vi "List Path Configurations.vi"(8 "error in (no error)":errorcluster, 11 "VISA resource name":refnum<visa-resource-name>) -> (0 "error out":errorcluster, 2 "Path Configuration Array":string[](array[string]), 3 "VISA resource name out":refnum<visa-resource-name>)   [LabVIEW 2018, in "Keysight PNA Series.lvlib"]
doc: "Returns a list of configuration names stored in the PNA."
uses:
  Keysight PNA Series.lvlib
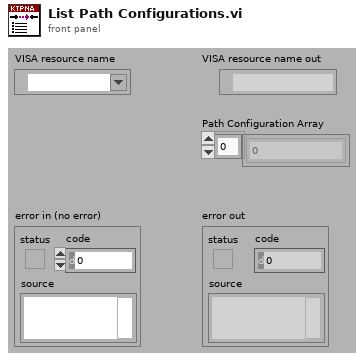
[diagram p1: front panel]
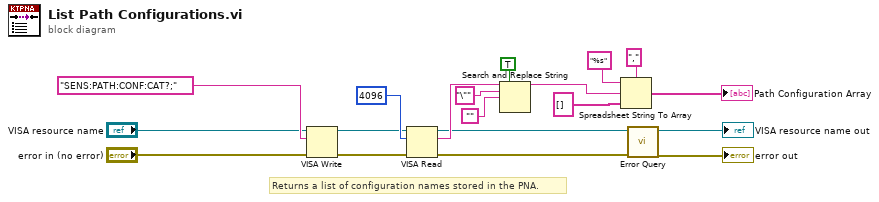
[diagram p0: block diagram]
diagram:
  # "Returns a list of configuration names stored in the PNA."
  n1 = VISA Write(VISA resource name="VISA resource name", write buffer="SENS:PATH:CONF:CAT?;", error in (no error)="error in (no error)") -> (VISA resource name out=w15:refnum<visa-resource-name>, error out=w14:errorcluster)  [unwired: 1 out]
  n2 = VISA Read(VISA resource name=w15, byte count=u32 4096, error in (no error)=w14) -> (VISA resource name out=w2:refnum<visa-resource-name>, read buffer=w3:string, error out=w4:errorcluster)  [unwired: 1 out]
  n3 = Search and Replace String(replace all?=TRUE ("replace all? (F)"), input string=w3, search string="\"", replace string="") -> (result string=w1:string)  [unwired: 4 in, 3 out]
  n4 = Spreadsheet String To Array(delimiter (Tab)=",", format string="%s", spreadsheet string=w1, array type (2D Dbl)=string[] []) -> (array=→"Path Configuration Array":string[])
  n5 = call "Error Query.vi"("error in (no error)"=w4, "VISA resource name"=w2) -> ("error out"=→"error out":errorcluster, "VISA resource name out"=→"VISA resource name out":refnum<visa-resource-name>)  [unwired: 6 in, 2 out]
